vi "test Passes If Arrays Are Equal And Comparison Is Non Case Sensitive.vi"(8 "error in (no error)":errorcluster, 11 "TestCase in":refnum<class "Pass If Equal 1D Array (String) Test Case.lvclass">) -> (0 "error out":errorcluster, 3 "TestCase out":refnum<class "Pass If Equal 1D Array (String) Test Case.lvclass">)   [LabVIEW 2015, in "Pass If Equal 1D Array (String) Test Case.lvclass"]
uses:
  Pass If Equal 1D Array (String) Test Case.lvclass
  <vilib>/addons/_JKI Toolkits/VI Tester/TestCase.llb/TestCase.lvclass
  VITAC.lvlib
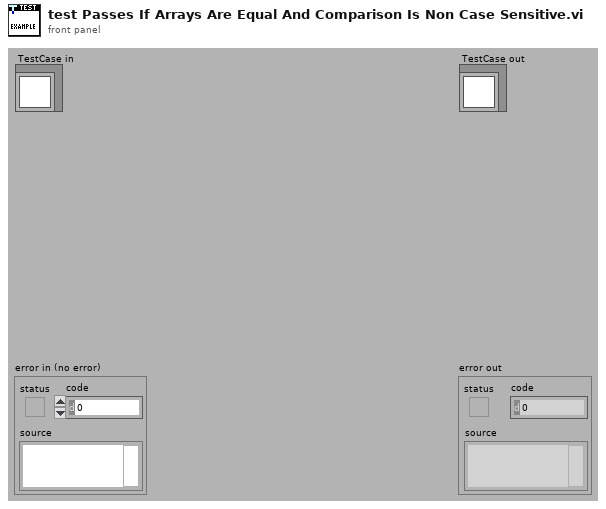
[diagram p1: front panel]
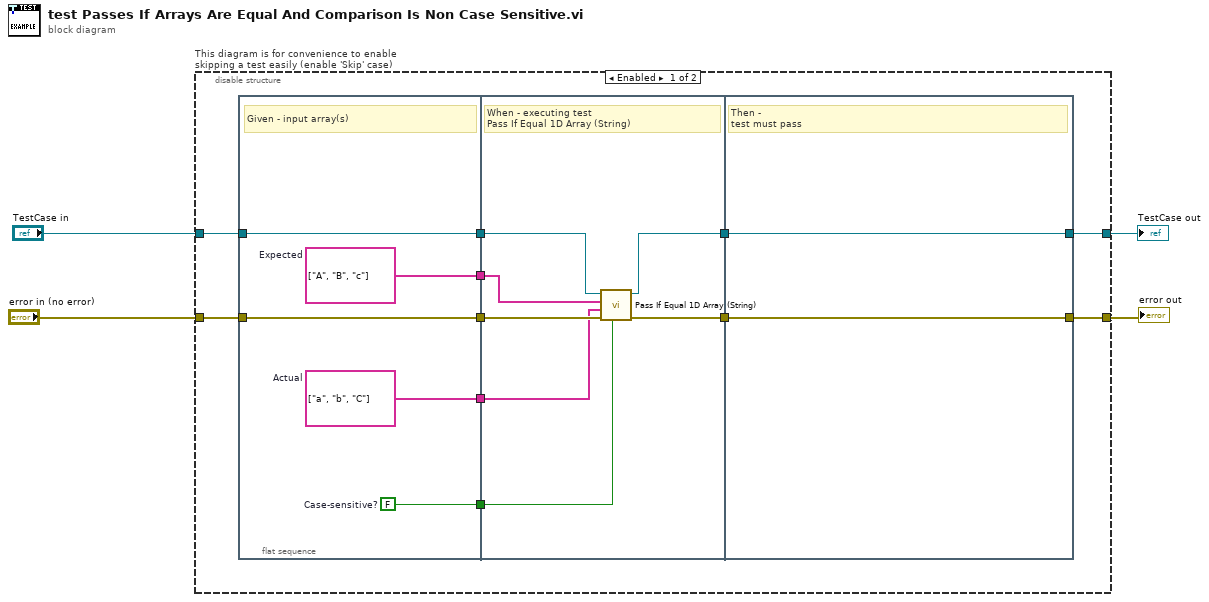
[diagram p0: block diagram]
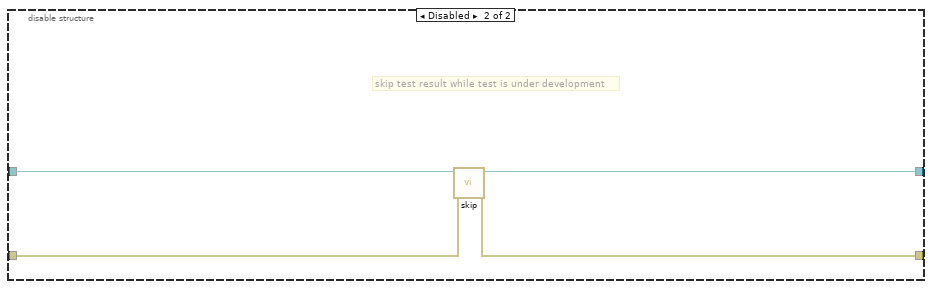
[diagram p2: hidden frame]
diagram:
  n1 = disable-structure "This diagram is for convenience to enable skipping a test easily (enable 'Skip' case)" shown="Enabled" {
    disable-tunnel: "TestCase in" -> [w12 w33]
    disable-tunnel: [w15 w31] -> w1
    disable-tunnel: [w11 w32] -> w3
    disable-tunnel: "error in (no error)" -> [w8 w30]
    frame Enabled {
      n2 = flat-sequence {
        tunnel: [w20] -> w13
        tunnel: w12 -> [w20]
        tunnel: [w19] -> w9
        tunnel: w8 -> [w19]
        tunnel: [w18] -> w7
        tunnel: [w17] -> w6
        tunnel: [w16] -> w5
        tunnel: [w24] -> w14
        tunnel: w13 -> [w25]
        tunnel: [w26] -> w10
        tunnel: w9 -> [w27]
        tunnel: w7 -> [w23]
        tunnel: w6 -> [w22]
        tunnel: w5 -> [w21]
        tunnel: [w29] -> w15
        tunnel: w14 -> [w29]
        tunnel: [w28] -> w11
        tunnel: w10 -> [w28]
        frame #0 {
          w18 = FALSE  # Case-sensitive?
          w17 = string[] ["a", "b", "C"]  # Actual
          w16 = string[] ["A", "B", "c"]  # Expected
          # "Given - input array(s)"
        }
        frame #1 {
          # "When - executing test \nPass If Equal 1D Array (String)"
          n3 = call "Pass If Equal 1D Array (String).vi"("case sensitive?"=w23, "error in (no error)"=w27, "actual"=w22, "expected"=w21, "TestCase in"=w25) -> ("error out"=w26:errorcluster, "TestCase out"=w24:refnum<class "Pass If Equal 1D Array (String) Test Case.lvclass">)  [unwired: 5 in]
        }
        frame #2 {
          # "Then - \ntest must pass"
        }
      }
    }
    frame Disabled {
      # "skip test result while test is under development"
      n4 = call <vilib>:"skip.vi"("error in (no error)"=w30, "TestCase in"=w33) -> ("error out"=w32:errorcluster, "TestCase out"=w31:refnum<class "Pass If Equal 1D Array (String) Test Case.lvclass">)  [unwired: 8 in]
    }
  }
  "error out" <- w3
  "TestCase out" <- w1
